vi "GetParam.vi"(8 "error in (no error)":errorcluster caption="entrée d'erreur (pas d'erreur)", 11 "FunctionTransformer.lvclass":refnum<class "FunctionTransformer.lvclass">) -> (0 "error out":errorcluster caption="sortie d'erreur", 2 "FunctionTransformer":T1={"func_callable"="None", "inverse_func_callable"="None", "validate"=FALSE, "accept_sparse"=FALSE, "check_inverse"=TRUE, "kw_args"={"key"=[], "Value"=[]}, "inv_kw_args"={"key"=[], "Value"=[]}}, 3 "FunctionTransformer.lvclass":refnum<class "FunctionTransformer.lvclass">)   [LabVIEW 2020, in "FunctionTransformer.lvclass"]
doc: "Get Parameters"
uses:
  FunctionTransformer.lvclass
  FunctionTransformer.lvclass/FunctionTransformer.ctl
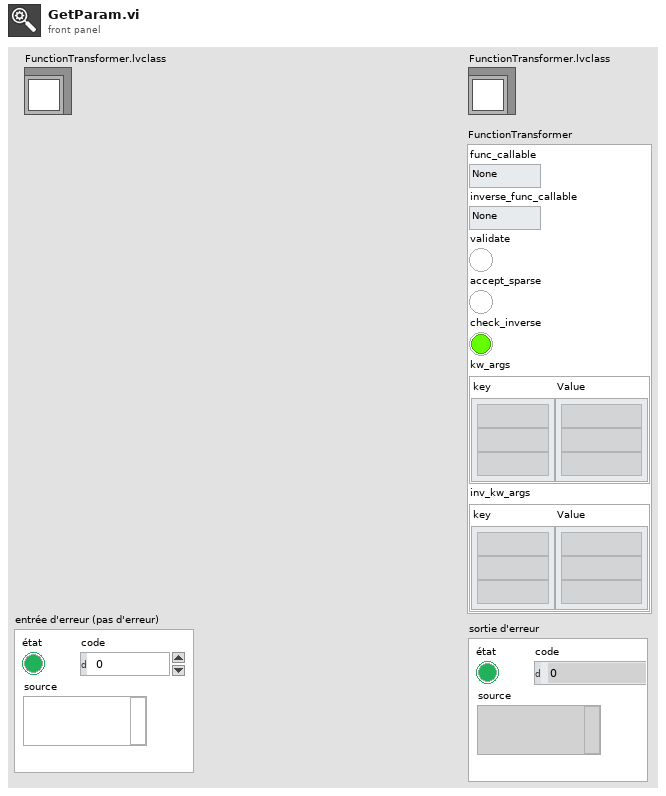
[diagram p1: front panel]
types:
  T1 = cluster{"func_callable":string, "inverse_func_callable":string, "validate":bool, "accept_sparse":bool, "check_inverse":bool, "kw_args":cluster{"key":string[], "Value":string[]}, "inv_kw_args":cluster{"key":string[], "Value":string[]}}
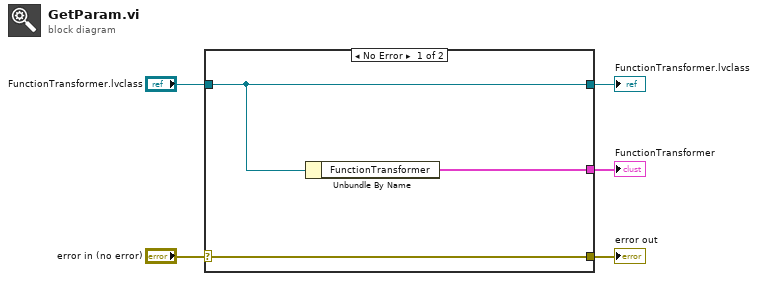
[diagram p0: block diagram]
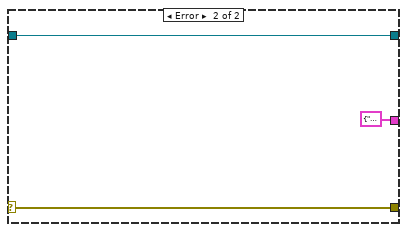
[diagram p2: hidden frame]
diagram:
  n1 = case shown="No Error" "error in (no error)" {
    selector: "error in (no error)" -> [w8 w10]
    tunnel: [w8 w10] -> w4
    tunnel: [w7 w11] -> w2
    tunnel: "FunctionTransformer.lvclass" -> [w7 w11]
    tunnel: [w6 T1 {"func_callable"="", "inverse_func_callable"="", "validate"=FALSE, "accept_sparse"=FALSE, "check_inverse"=FALSE, "kw_args"={"key"=[], "Value"=[]}, "inv_kw_args"={"key"=[], "Value"=[]}} ("FunctionTransformer")] -> w1
    frame No Error {
      n2 = Unbundle By Name(w7) -> ("FunctionTransformer"=w6:T1)
    }
    frame Error {
    }
  }
  "error out" <- w4
  "FunctionTransformer.lvclass" <- w2
  "FunctionTransformer" <- w1
